vi "QueueGlobal.vi"(6 "cmd (Add)":enum16{"Add One to End", "Get All", "Reset"}(ring), 8 "error in (no error)":errorcluster, 11 "queue name":string) -> (0 "error out":errorcluster, 3 "queue names":string[](array[string]))   [LabVIEW 2009]
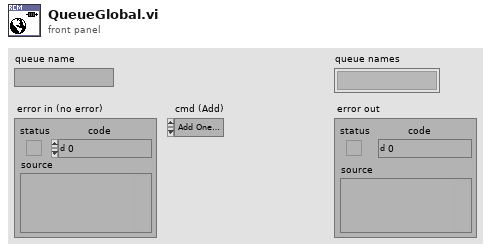
[diagram p1: front panel]
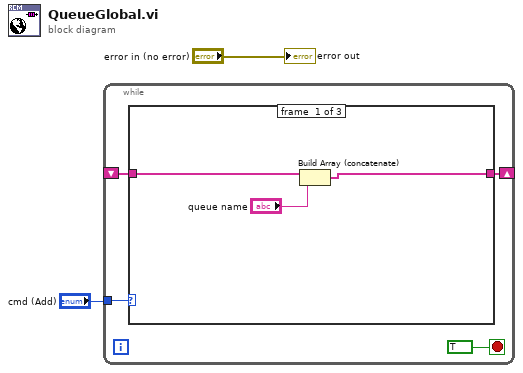
[diagram p0: block diagram]
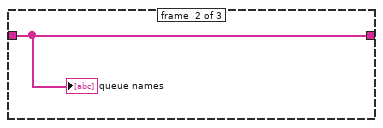
[diagram p2: hidden frame]
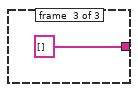
[diagram p3: hidden frame]
diagram:
  n1 = while {
    tunnel: "cmd (Add)" -> [w5]
    shift-right: [w4] -> _
    shift-left: _ -> [w3]
    stop <- TRUE stop-if-true
    n2 = case shown="\"Get All\"" w5 {
      tunnel: [w8 w10 string[] []] -> w4
      tunnel: w3 -> [w9 w10 _]
      frame #0 {
        n3 = Build Array (concatenate)(w9, "queue name") -> (w8:string[])
      }
      frame #1 {
        "queue names" <- w10
      }
      frame #2 {
      }
    }
  }
  "error out" <- "error in (no error)"
